vi "close connection.vi"(8 "error in (no error)":errorcluster, 11 "MB in":refnum<class "Modbus Master CR.lvclass">) -> (0 "error out":errorcluster, 3 "MB out":refnum<class "Modbus Master CR.lvclass">)   [LabVIEW 2021, in "Modbus Master CR.lvclass"]
uses:
  Modbus Master CR.lvclass
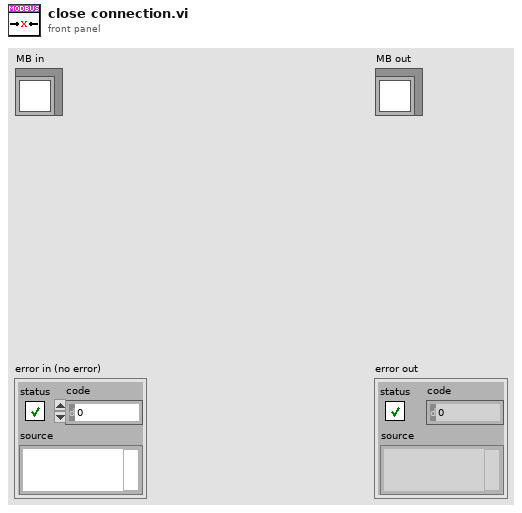
[diagram p1: front panel]
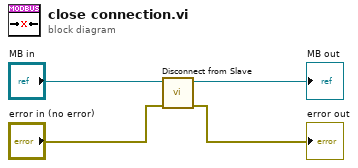
[diagram p0: block diagram]
diagram:
  n1 = call-dynamic "Disconnect from Slave.vi"("error in (no error)"="error in (no error)", "network master in"="MB in") -> ("error out"=→"error out":errorcluster, "network master out"=→"MB out":refnum<class "Modbus Master CR.lvclass">)  [unwired: 8 in]
